vi "P03_Formula General - String.vi"() -> ()   [LabVIEW 2026]
panel:
  out "Ecuación insertada":string
  out "Tipo de  raíz":string
  out "XY Graph":cluster{dbl[], dbl[]}(graph)
  in  "stop":bool
  out "Warning":string
  out "X2":string
  out "X1":string
  in  "CALCULAR":bool
  in  "C":dbl
  in  "B":dbl
  in  "A":dbl
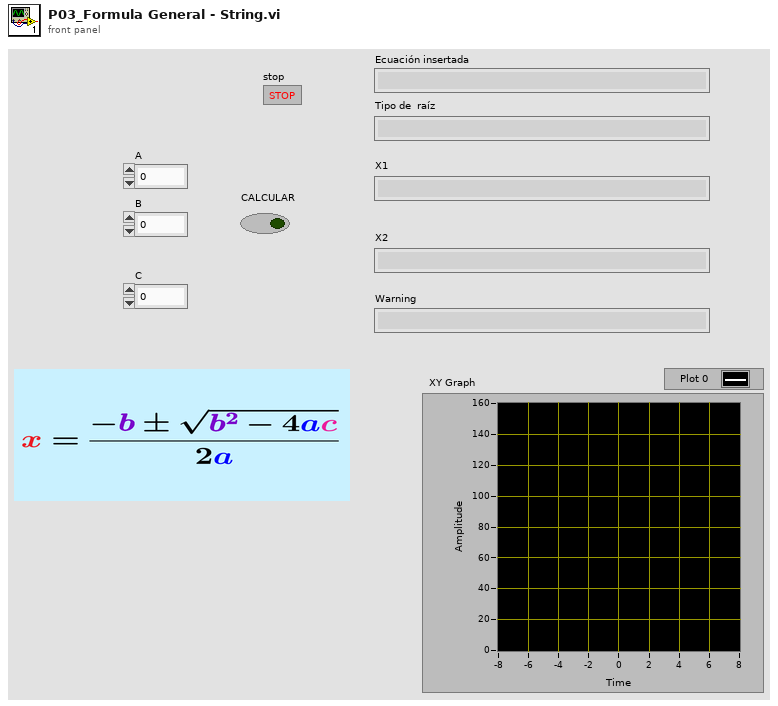
[diagram p1: front panel]
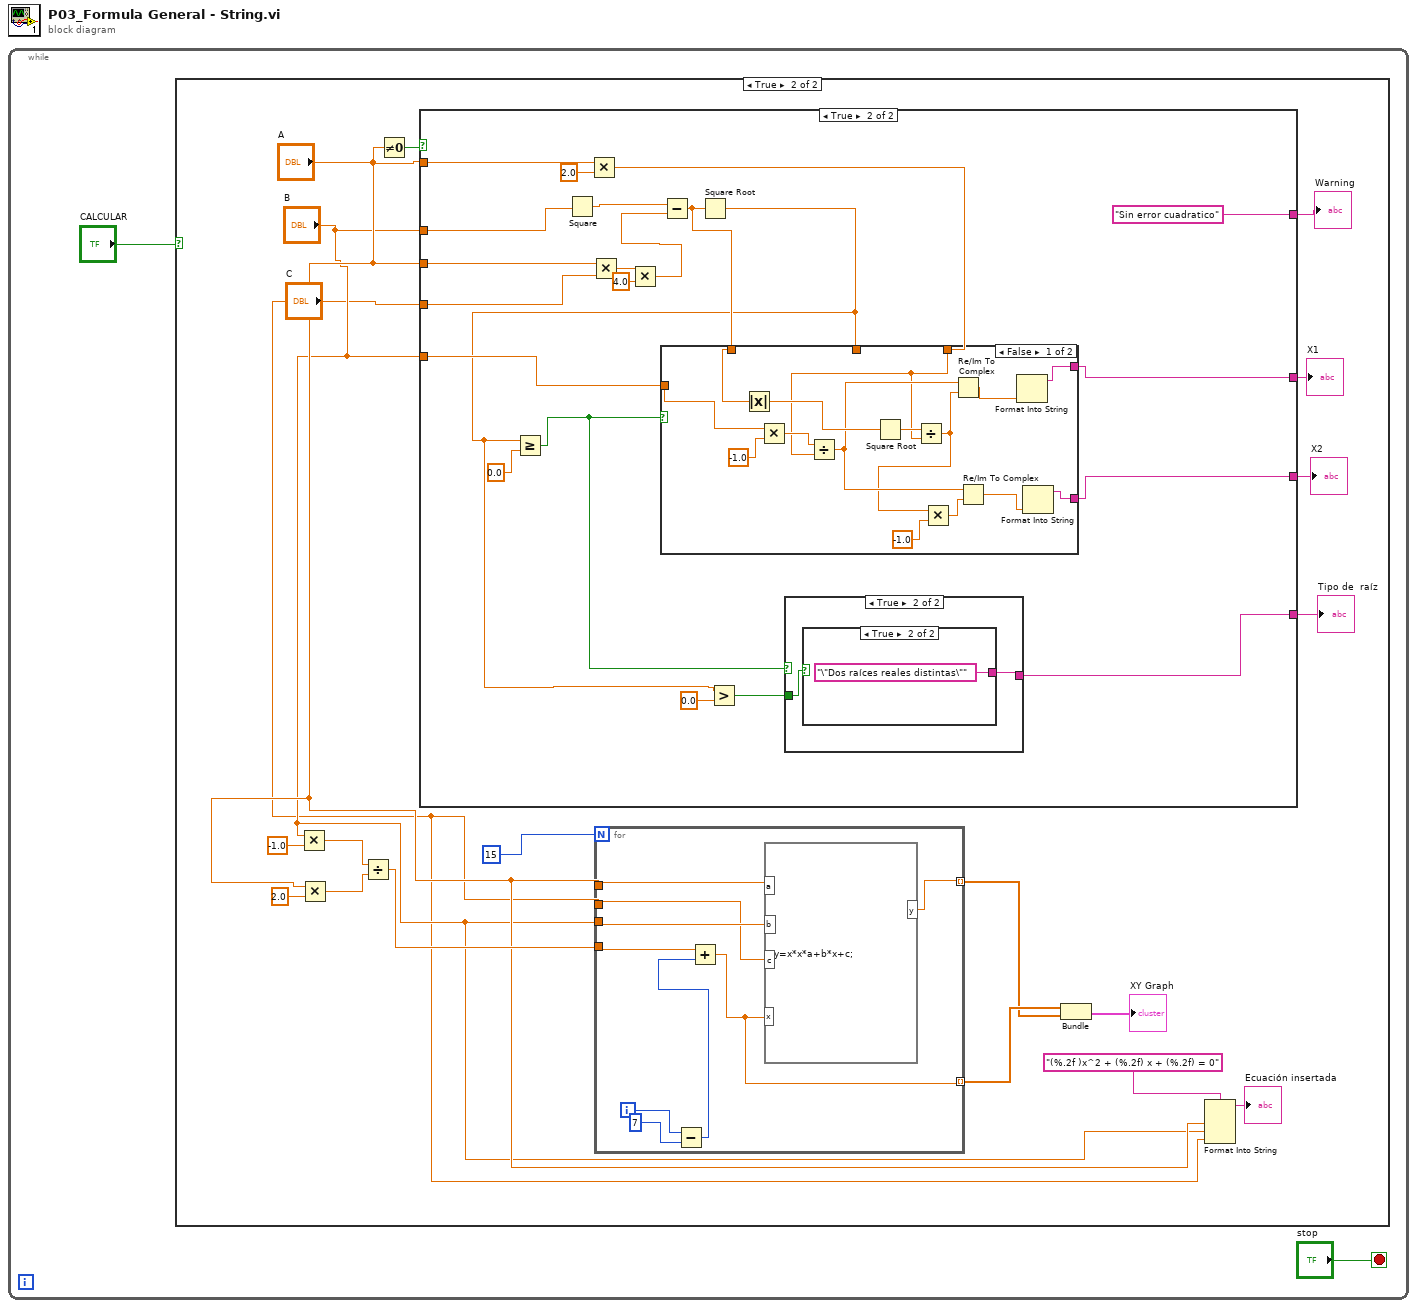
[diagram p0: block diagram]
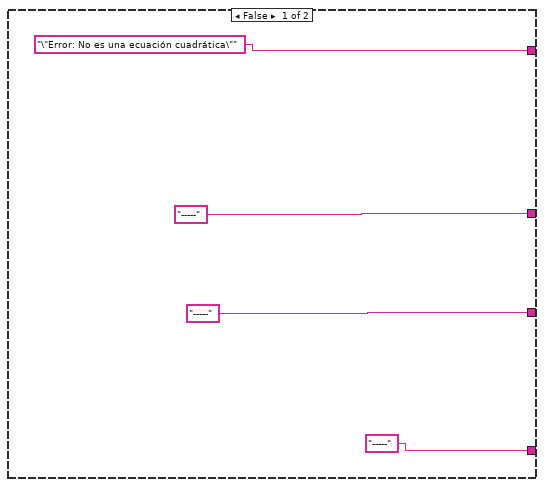
[diagram p3: hidden frame]
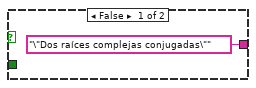
[diagram p4: hidden frame]
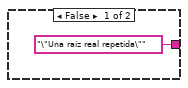
[diagram p5: hidden frame]
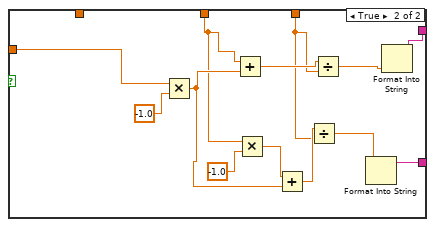
[diagram p6: hidden frame]
diagram:
  n1 = while {
    stop <- "stop" stop-if-true
    n2 = case shown="True" "CALCULAR" {
      frame False {
      }
      frame True {
        n3 = Multiply(x="B", y=-1.0) -> (x*y=w19:dbl)
        n4 = Multiply(x="A", y=2.0) -> (x*y=w18:dbl)
        n5 = Divide(x=w19, y=w18) -> (x/y=w14:dbl)
        n6 = Not Equal To 0?(x="A") -> (x != 0?=w21:bool)
        n7 = case shown="True" w21 {
          tunnel: "B" -> [_ w55]
          tunnel: "A" -> [_ w54]
          tunnel: "C" -> [_ w53]
          tunnel: "B" -> [_ w44]
          tunnel: "A" -> [_ w48]
          tunnel: ["\"Error: No es una ecuación cuadrática\"" ("Warning") "Sin error cuadratico" ("Warning")] -> w20
          tunnel: ["-----" w41] -> w10
          tunnel: ["-----" w40] -> w9
          tunnel: ["-----" w38] -> w8
          frame False {
          }
          frame True {
            n8 = Square(x=w55) -> (x^2=w49:dbl)
            n9 = Multiply(x=w48, y=2.0) -> (x*y=w45:dbl)
            n10 = Multiply(x=w54, y=w53) -> (x*y=w52:dbl)
            n11 = Multiply(x=w52, y=4.0) -> (x*y=w50:dbl)
            n12 = Subtract(x=w49, y=w50) -> (x-y=w42:dbl)
            n13 = Square Root(x=w42) -> (sqrt(x)=w36:dbl)
            n14 = Greater Or Equal?(x=w36, y=0.0) -> (x >= y?=w39:bool)
            n15 = case shown="False" w39 {
              tunnel: w45 -> [w61 w84]
              tunnel: w36 -> [_ w77]
              tunnel: [w74 w83] -> w40
              tunnel: [w75 w82] -> w41
              tunnel: w44 -> [w69 w80]
              tunnel: w42 -> [w71 _]
              frame False {
                n16 = Absolute Value(x=w71) -> (abs(x)=w70:dbl)
                n17 = Multiply(x=w69, y=-1.0) -> (x*y=w65:dbl)
                n18 = Divide(x=w65, y=w61) -> (x/y=w64:dbl)
                n19 = Square Root(x=w70) -> (sqrt(x)=w62:dbl)
                n20 = Divide(x=w62, y=w61) -> (x/y=w63:dbl)
                n21 = Multiply(x=w63, y=-1.0) -> (x*y=w66:dbl)
                n22 = Re/Im To Complex(1:w63, 2:w64) -> (0:w73:cdb)
                n23 = Re/Im To Complex(1:w66, 2:w64) -> (0:w72:cdb)
                n24 = Format Into String(w73) -> (resulting string=w75:string)  [unwired: 3 in, 1 out]
                n25 = Format Into String(w72) -> (resulting string=w74:string)  [unwired: 3 in, 1 out]
              }
              frame True {
                n26 = Multiply(x=w80, y=-1.0) -> (x*y=w79:dbl)
                n27 = Add(x=w77, y=w79) -> (x+y=w85:dbl)
                n28 = Multiply(x=w77, y=-1.0) -> (x*y=w76:dbl)
                n29 = Add(x=w76, y=w79) -> (x+y=w86:dbl)
                n30 = Divide(x=w86, y=w84) -> (x/y=w88:dbl)
                n31 = Divide(x=w85, y=w84) -> (x/y=w87:dbl)
                n32 = Format Into String(w88) -> (resulting string=w83:string)  [unwired: 3 in, 1 out]
                n33 = Format Into String(w87) -> (resulting string=w82:string)  [unwired: 3 in, 1 out]
              }
            }
            n34 = Greater?(x=w36, y=0.0) -> (0:w35:bool)
            n35 = case shown="True" w39 {
              tunnel: ["\"Dos raíces complejas conjugadas\"" w57] -> w38
              tunnel: w35 -> [_ w58]
              frame False {
              }
              frame True {
                n36 = case shown="True" w58 {
                  tunnel: ["\"Una raíz real repetida\"" "\"Dos raíces reales distintas\""] -> w57
                  frame False {
                  }
                  frame True {
                  }
                }
              }
            }
          }
        }
        "Warning" <- w20
        "X1" <- w10
        "X2" <- w9
        "Tipo de  raíz" <- w8
        n37 = for {
          N: 15 -> [_]
          tunnel: w14 -> [w28]
          tunnel: "A" -> [w26]
          tunnel: "B" -> [w25]
          tunnel: "C" -> [w24]
          tunnel: [w23] -> w13 mode=indexing
          tunnel: [w22] -> w12 mode=indexing
          i -> [w30]
          n38 = Subtract(x=w30, y=7) -> (x-y=w27:i32)
          n39 = Add(x=w28, y=w27) -> (x+y=w23:dbl)
          n40 = formula code="y=x*x*a+b*x+c;"("x"=w23, "a"=w26, "b"=w25, "c"=w24) -> ("y"=w22:dbl)
        }
        n41 = Bundle(w13, w12) -> (→"XY Graph":cluster{dbl[], dbl[]})  [unwired: 1 in]
        n42 = Format Into String(format string="(%.2f )x^2 + (%.2f) x + (%.2f) = 0", "A", "B", "C") -> (resulting string=→"Ecuación insertada":string)  [unwired: 2 in, 1 out]
      }
    }
  }
